vi "lvlibp_FD_Strings.vi"() -> ()   [LabVIEW 2016]
panel:
  in  "drive not exist":string="无法读取驱动器%s，再试一次？" caption="驱动器不存在"
  in  "file not exist":string=" 不存在。" caption="文件不存在"
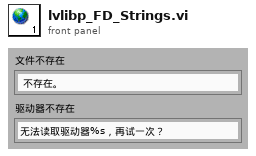
[diagram p1: front panel]
diagram:
